vi "Launcher.vi"() -> ()   [LabVIEW 2019]
uses:
  UI Actor.lvclass
  C:/Program Files/National Instruments/LabVIEW 2019/vi.lib/ActorFramework/Actor/Actor.lvclass
  UI Actor.lvclass/UI Actor.ctl
  Write Monedas.vi
  Write Productos.vi
  Write Idioma.vi
  <vilib>/ActorFramework/Actor/Actor.lvclass
panel:
  in  "Idioma":enum16{"Español", "Ingles"}(ring)
  in  "Productos":enum16{"Coca", "Nestle"}(ring)
  in  "Monedas":enum16{"MXN", "USD"}(ring)
  in  "error in (no error)":errorcluster
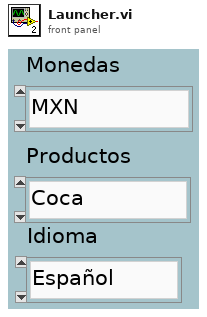
[diagram p1: front panel]
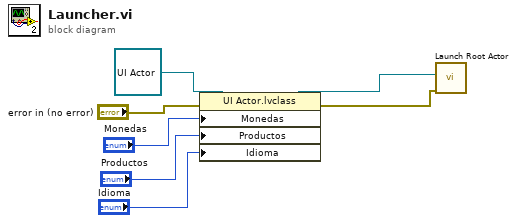
[diagram p0: block diagram]
diagram:
  n1 = property class="UI Actor.lvclass"(reference=refnum<class "UI Actor.lvclass"> refnum ("UI Actor.lvlib:UI Actor.lvclass"), error in="error in (no error)", "Monedas"="Monedas", "Productos"="Productos", "Idioma"="Idioma") -> (reference out=w7:refnum<class "UI Actor.lvclass">, error out=w5:errorcluster)
  n2 = call <vilib>:"Launch Root Actor.vi"("error in (no error)"=w5, "Actor"=w7) -> ()  [unwired: 8 in, 2 out]
